vi "GLBL_9403_DIO_0_31.vi"(10 "9403_DIO":T1, 11 "write_read":bool) -> (2 "9403_DIO out":T1)   [LabVIEW 2020]
uses:
  controls/DIO_0_31.ctl
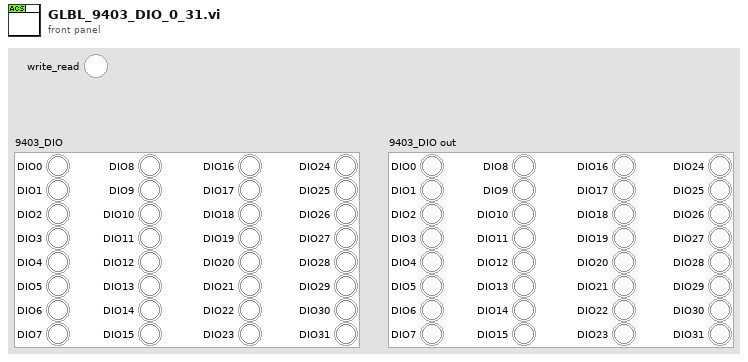
[diagram p1: front panel]
types:
  T1 = typedef "DIO_0_31.ctl" = cluster{"DIO0":bool, "DIO1":bool, "DIO2":bool, "DIO3":bool, "DIO4":bool, "DIO5":bool, "DIO6":bool, "DIO7":bool, "DIO8":bool, "DIO9":bool, "DIO10":bool, "DIO11":bool, "DIO12":bool, "DIO13":bool, "DIO14":bool, "DIO15":bool, "DIO16":bool, "DIO17":bool, "DIO18":bool, "DIO19":bool, "DIO20":bool, "DIO21":bool, "DIO22":bool, "DIO23":bool, "DIO24":bool, "DIO25":bool, "DIO26":bool, "DIO27":bool, "DIO28":bool, "DIO29":bool, "DIO30":bool, "DIO31":bool}
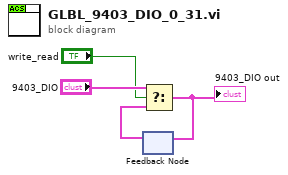
[diagram p0: block diagram]
diagram:
  n1 = feedback #1() -> (w3:T1)  [unwired: 1 in]
  n2 = Select(t="9403_DIO", s="write_read", f=w3) -> (s? t:f=w2:T1)
  "9403_DIO out" <- w2
  n3 = feedback-in #1(w2) -> ()
